vi "Wait for finish.vi"(8 "error in (no error)":errorcluster, 9 "timeout in ms (-1)":i32=-1, 11 "Process In":refnum<class "Process.lvclass">) -> (0 "error out":errorcluster, 1 "timed out?":bool, 3 "Process Out":refnum<class "Process.lvclass">)   [LabVIEW 2020, in "Process.lvclass"]
uses:
  Process.lvclass
  Process.lvclass/Process.ctl
  <vilib>/Utility/error.llb/Error Cluster From Error Code.vi
  <vilib>/ErrorRing/Error Ring.xnode
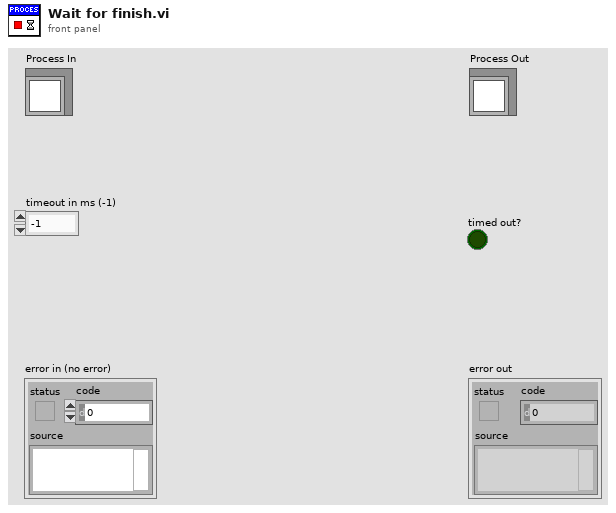
[diagram p1: front panel]
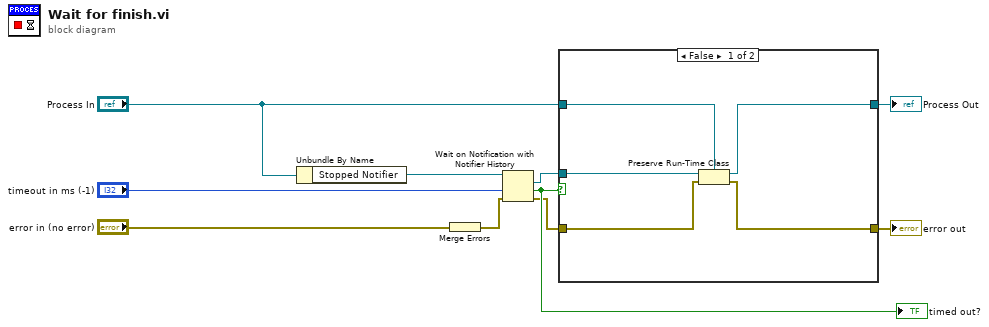
[diagram p0: block diagram]
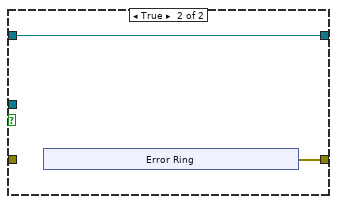
[diagram p2: hidden frame]
diagram:
  n1 = Unbundle By Name("Process In") -> ("Stopped Notifier"=w10:refnum<notifier>)
  n2 = Merge Errors("error in (no error)") -> (w1:errorcluster)
  n3 = Wait on Notification with Notifier History(0:w10, 2:"timeout in ms (-1)", 3:w1) -> (9:w4:refnum<class "Base.lvclass">, 10:w6:bool, 11:w5:errorcluster)  [unwired: 1 in, 1 out]
  "timed out?" <- w6
  n4 = case shown="False" w6 {
    tunnel: [w13 w17] -> w7
    tunnel: w5 -> [w12 _]
    tunnel: w4 -> [w15 _]
    tunnel: [w11 w16] -> w3
    tunnel: "Process In" -> [w14 w16]
    frame False {
      n5 = Preserve Run-Time Class(object in=w15, error in=w12, 2:w14) -> (object out=w11:refnum<class "Process.lvclass">, error out=w13:errorcluster)
    }
    frame True {
      n6 = xnode "Error Ring"() -> ("error out"=w17:errorcluster)
    }
  }
  "error out" <- w7
  "Process Out" <- w3
